vi "S2C_UTILITY_Proc_CntPrompt.vi"(8 "Error In":errorcluster, 11 "Message":string) -> (0 "Error Out":errorcluster, 3 "Cnt":i32)   [LabVIEW 2015]
panel:
  out "Init":bool
  in  "Done":bool
  in  "Count":i32
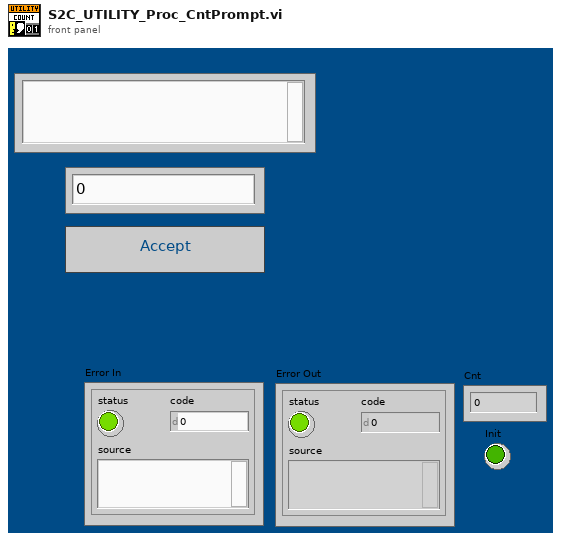
[diagram p1: front panel]
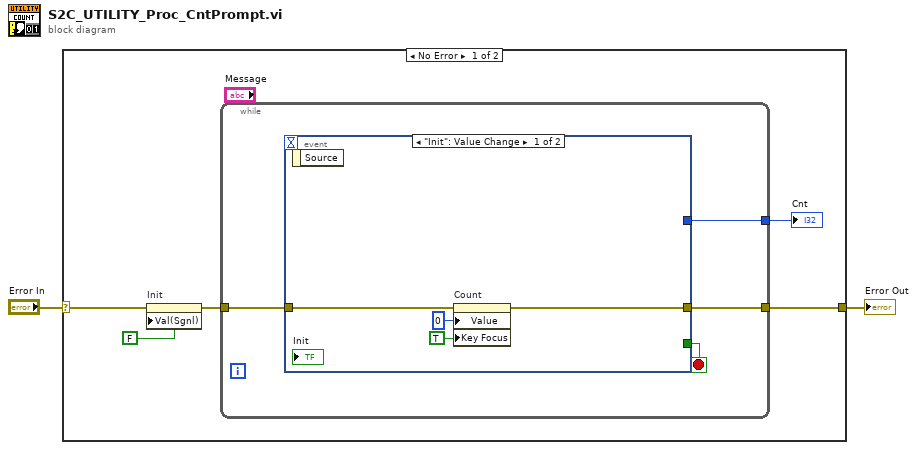
[diagram p0: block diagram]
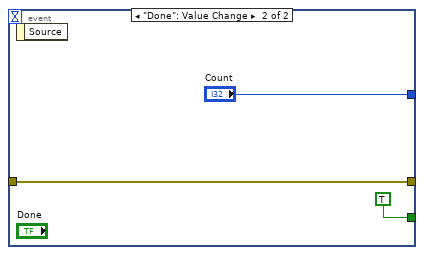
[diagram p2: hidden frame]
diagram:
  n1 = case shown="No Error" "Error In" {
    selector: "Error In" -> [w5 w19]
    tunnel: [w7 w19] -> w1
    frame No Error {
      n2 = property on="Init" class="Bool (strict)"(error in=w5, "Val(Sgnl)"=FALSE ("Value (Signaling)")) -> (error out=w4:errorcluster)  [unwired: 1 in, 1 out]
      n3 = while {
        tunnel: w4 -> [w11]
        tunnel: [w10] -> w7
        tunnel: [w8] -> w6
        stop <- w9 stop-if-true
        n4 = event shown="[0] \"Init\": Value Change" {
          selector: _ -> [_ _]
          dyn-events: _ -> [_ _]
          timeout: _ -> [_ _]
          tunnel: w11 -> [w15 w18]
          tunnel: [w14 w18] -> w10
          tunnel: [_ TRUE] -> w9
          tunnel: [_ "Count"] -> w8
          event "Init": Value Change {
            n5 = event-data() -> ()  [unwired: 1 in, 1 out]
            n6 = property on="Count" class="DigNum (strict)"(error in=w15, "Value"=0 ("Count"), "Key Focus"=TRUE) -> (error out=w14:errorcluster)  [unwired: 1 in, 1 out]
          }
          event "Done": Value Change {
            n7 = event-data() -> ()  [unwired: 1 in, 1 out]
          }
        }
      }
      "Cnt" <- w6
    }
    frame Error {
    }
  }
  "Error Out" <- w1
